vi "Write.vi"(8 "error in (no error)":errorcluster, 10 "Data To Write":string, 11 "Network Interface":refnum<data-value>) -> (0 "error out":errorcluster, 3 "Network Interface Out":refnum<data-value>)   [LabVIEW 2017, in "Network Interface.lvlib" / "Network Interface.lvclass"]
uses:
  <vilib>/gpm_packages/@cs/Network-Sink/Source/Network Interface/Network Interface/Network Interface.lvclass
  <vilib>/gpm_packages/@cs/Network-Sink/Source/Network Interface/Connection Handler/Synchronous Write Request.ctl
  <vilib>/gpm_packages/@cs/Network-Sink/Source/Network Interface/Network Session Handler/Session Handler Message Names ENUM.ctl
  <vilib>/gpm_packages/@cs/Network-Sink/Source/Network Interface/Network Interface/Network Interface.lvclass/Network Interface.ctl
  <vilib>/gpm_packages/@cs/Network-Sink/Source/Network Interface/Message Queue/Message Queue.lvclass/Message Queue.ctl
  dc351019-4f29-47b2-a483-8ae26d0321a6.vi
  <vilib>/gpm_packages/@cs/Network-Sink/Source/Network Interface/Message Queue/Protected Enqueue.vi
  <vilib>/gpm_packages/@cs/Network-Sink/Source/Network Interface/Connection Handler/Connection Handler.lvclass
  <vilib>/gpm_packages/@cs/Network-Sink/Source/Network Interface/Network Session Handler/Network Session Handler.lvclass
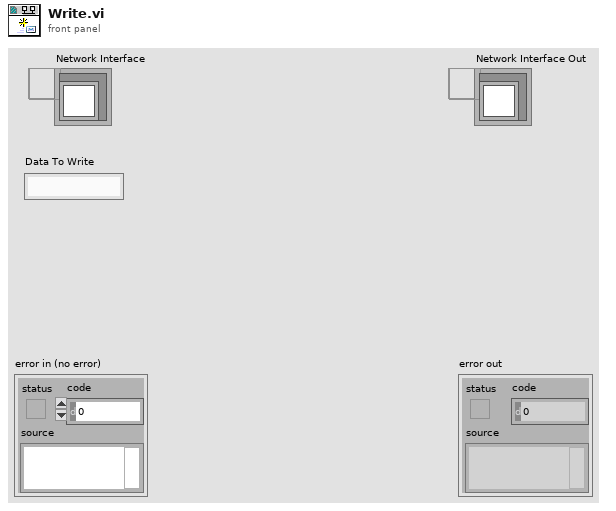
[diagram p1: front panel]
types:
  T1 = typedef "Network Interface.lvlib/Network Session Handler.lvclass/Session Handler Message Names ENUM.ctl" = enum16{"Transmit Message", "Stop", "Handler Shutdown", "Error"}
  T2 = typedef "Network Interface.lvlib/Connection Handler.lvclass/Synchronous Write Request.ctl" = cluster{"Data To Write":string, "Return Queue":refnum<queue>}
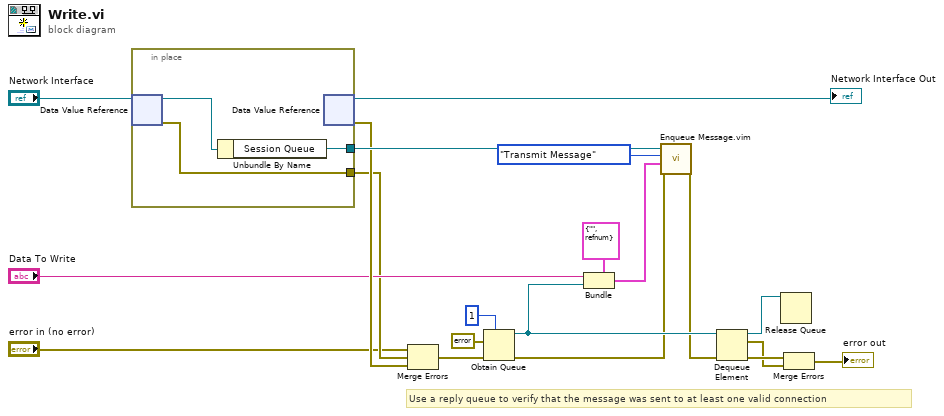
[diagram p0: block diagram]
diagram:
  # "Use a reply queue to verify that the message was sent to at least one valid connection"
  n1 = in-place {
    in-place-border: [w22] -> w11
    in-place-border: [w21] -> w2
    n2 = in-place-dvr #1("Network Interface") -> (w23:refnum<class "Network Interface.lvclass">, w21:errorcluster)
    n3 = Unbundle By Name(w23) -> ("Session Queue"=w22:refnum<class "Message Queue.lvclass">)
    n4 = in-place-dvr #1() -> (→"Network Interface Out":refnum<data-value>, w7:errorcluster)  [unwired: 1 in]
  }
  n5 = Merge Errors("error in (no error)", w2, w7) -> (w5:errorcluster)
  n6 = Obtain Queue(max queue size (-1, unlimited)=1, element data type=errorcluster {"status"=FALSE, "code"=0, "source"=""} ("error in (no error)"), error in (no error)=w5) -> (queue out=w12:refnum<queue>, error out=w4:errorcluster)  [unwired: 2 in, 1 out]
  n7 = Bundle(cluster=T2 {"Data To Write"="", "Return Queue"=refnum} ("output cluster"), "Data To Write"="Data To Write", "Return Queue"=w12) -> (w10:T2)
  n8 = call "Enqueue Message.vim"("error in (no error)"=w4, "Data"=w10, "Msg"=Session_Handler_Message_Names_ENUM."Transmit Message" ("Session Handler Messages"), "Message Queue in"=w11) -> ("error out"=w6:errorcluster)  [unwired: 6 in, 1 out]
  n9 = Dequeue Element(queue=w12, error in (no error)=w6) -> (queue out=w14:refnum<queue>, element=w16:errorcluster, error out=w17:errorcluster)  [unwired: 1 in, 1 out]
  n10 = Release Queue(queue=w14) -> ()  [unwired: 2 in, 3 out]
  n11 = Merge Errors(w17, w16) -> (→"error out":errorcluster)
